vi "todB.vi"(1 "Entrada [V]":dbl) -> (0 "Salida [dB]":dbl)   [LabVIEW 2018]
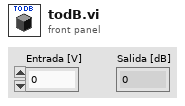
[diagram p1: front panel]
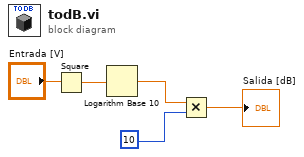
[diagram p0: block diagram]
diagram:
  n1 = Square(x="Entrada [V]") -> (x^2=w2:dbl)
  n2 = Logarithm Base 10(1:w2) -> (0:w5:dbl)
  n3 = Multiply(x=w5, y=10) -> (x*y=→"Salida [dB]":dbl)
